vi "Turbo_Encode.vi"(4 "cdblkseg_data_DL":dbl[][](array[numeric]), 5 "CpKpCmKmF":T1, 6 "error in (no error)":errorcluster caption="错误输入（无错误）", 7 "appended path":path) -> (0 "error out":errorcluster caption="错误输出", 2 "Array":dbl[][](array[numeric]))   [LabVIEW 2015]
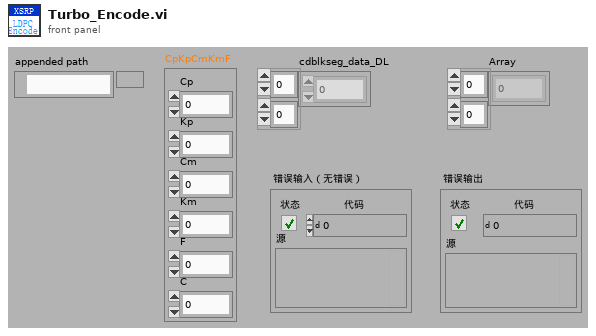
[diagram p1: front panel]
types:
  T1 = cluster{"Cp":dbl, "Kp":dbl, "Cm":dbl, "Km":dbl, "F":dbl, "C":dbl}
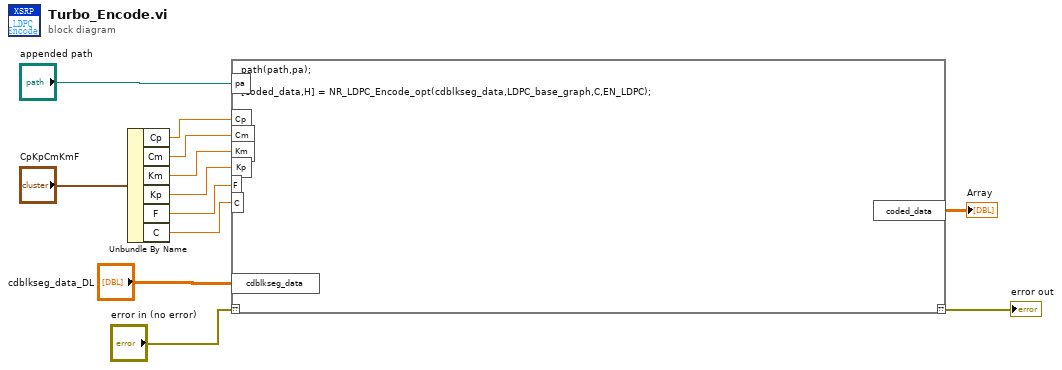
[diagram p0: block diagram]
diagram:
  n1 = Unbundle By Name("CpKpCmKmF") -> ("Cp"=w9:dbl, "Cm"=w8:dbl, "Km"=w7:dbl, "Kp"=w6:dbl, "F"=w5:dbl, "C"=w12:dbl)
  n2 = script code="path(path,pa);\n\n[coded_data,H] = NR_LDPC_Encode_opt(cdblkseg_data,LDPC_base_graph,C,EN_LDPC);"("??"="error in (no error)", "pa"="appended path", "Cp"=w9, "Cm"=w8, "cdblkseg_data"="cdblkseg_data_DL", "Km"=w7, "Kp"=w6, "F"=w5, "C"=w12) -> ("??"=→"error out":errorcluster, "coded_data"=→"Array":dbl[][])
